vi "CRYAdd rep #s to results headers.vi"(11 "Result array in":T1 {"Margin" format="%.2f"}) -> (3 "Result array with rep #'s":T1 {"Margin" format="%.2f"})   [LabVIEW 2013]
uses:
  Typedef Control/CRYResult Cluster Array.ctl
  Typedef Control/CRYResult Cluster.ctl
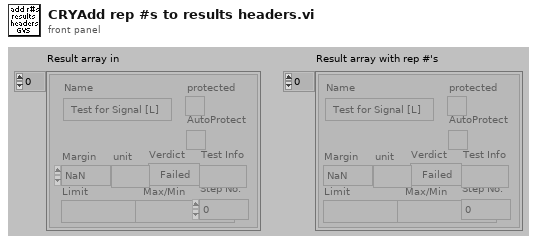
[diagram p1: front panel]
types:
  T1 = typedef "CRYResult Cluster Array.ctl" = T2[]
  T2 = typedef "CRYResult Cluster.ctl" = cluster{"Name":string, "Margin":dbl, "unit":string, "Verdict":bool, "Limit":string, "Max/Min":string, "protected":bool, "Step No.":i32, "Test Info":string, "AutoProtect":bool}
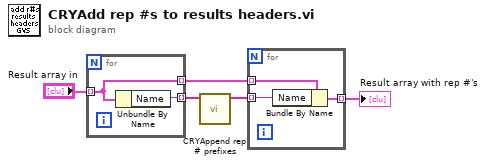
[diagram p0: block diagram]
diagram:
  n1 = for {
    tunnel: [w7] -> w5 mode=indexing
    tunnel: [w6] -> w3 mode=indexing
    tunnel: "Result array in" -> [w6] mode=indexing
    n2 = Unbundle By Name(w6) -> ("Name"=w7:string)
  }
  n3 = call "CRYAppend rep # prefixes.vi"("Curves list in"=w5) -> ("Curves list with no repeats"=w4:string[])  [unwired: 10 out]
  n4 = for {
    tunnel: w4 -> [w9] mode=indexing
    tunnel: w3 -> [w10] mode=indexing
    tunnel: [w8] -> w1 mode=indexing
    n5 = Bundle By Name(cluster=w10, "Name"=w9) -> (w8:T2)
  }
  "Result array with rep #'s" <- w1
